vi "STICK_house.vi"() -> ()   [LabVIEW 2014]
panel:
  out "Temperature in Volts [V]":dbl format="%#_4g"
  out "On/Off":bool
  out "Error out":errorcluster
  out "P1":T1
  out "P2":T2
  out "Device ID":string
  in  "VISA resource name":refnum<visa-resource-name>
  out "Error":bool
  in  "Thermostat ON/OFF":bool=TRUE
  out "Happiness [%]":dbl(slide) scale=0.0..100.0
  out "Status":string="Water frozen!"
  out "Thermostat [°C]":dbl=20.0
  out "Outdoor temp":dbl(slide) scale=-20.0..40.0
  out "Time":timestamp format="%<%H:%M>T"
  out "Boiler temp":dbl(knob) max=60.0 scale=0.0..100.0
  out "Room temp":dbl(slide) scale=0.0..40.0
  out "Room [°C]":dbl format="%#_3g"
  out "Heat":bool
  out "?":T3(graph)
  in  "Stop Button":bool
  # "System values"
  # "Thermostat"
  # "Boiler"
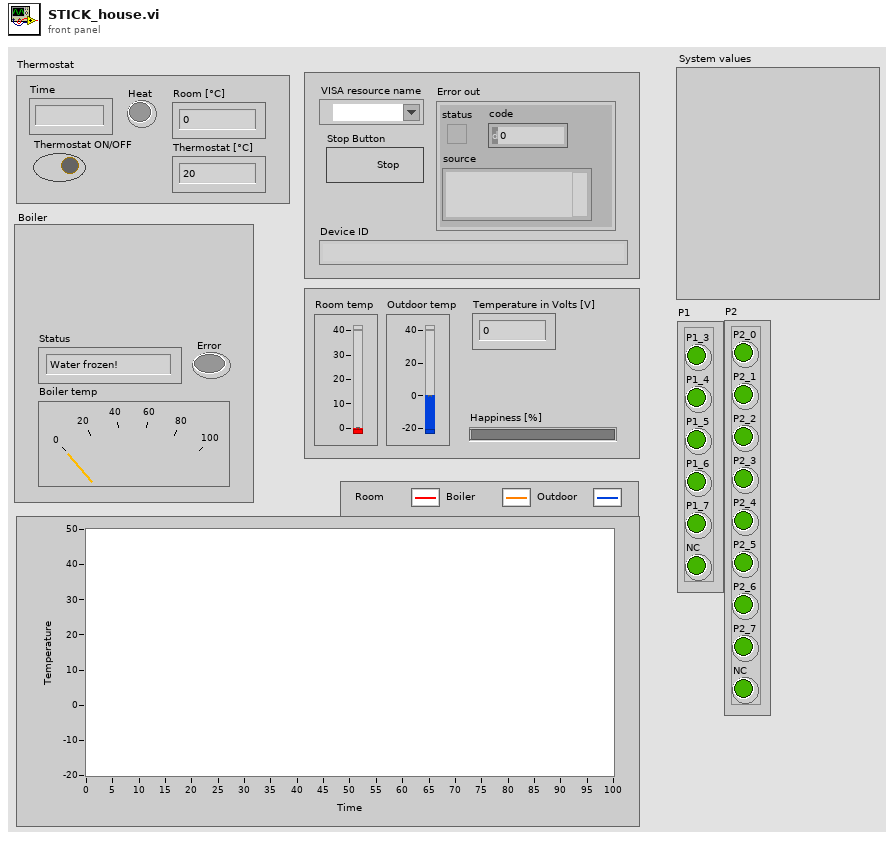
[diagram p1: front panel]
types:
  T1 = cluster{"P1_0":bool, "P1_1":bool, "P1_2":bool, "P1_3":bool, "P1_4":bool, "P1_5":bool, "P1_6":bool, "P1_7":bool, "NC":bool}
  T2 = cluster{"P2_0":bool, "P2_1":bool, "P2_2":bool, "P2_3":bool, "P2_4":bool, "P2_5":bool, "P2_6":bool, "P2_7":bool, "NC":bool}
  T3 = cluster{"T_room":dbl, "T_heater":dbl, "temp out":dbl}
  T4 = cluster{"T_room":dbl, "T_heater":dbl, "temp out":dbl}[]
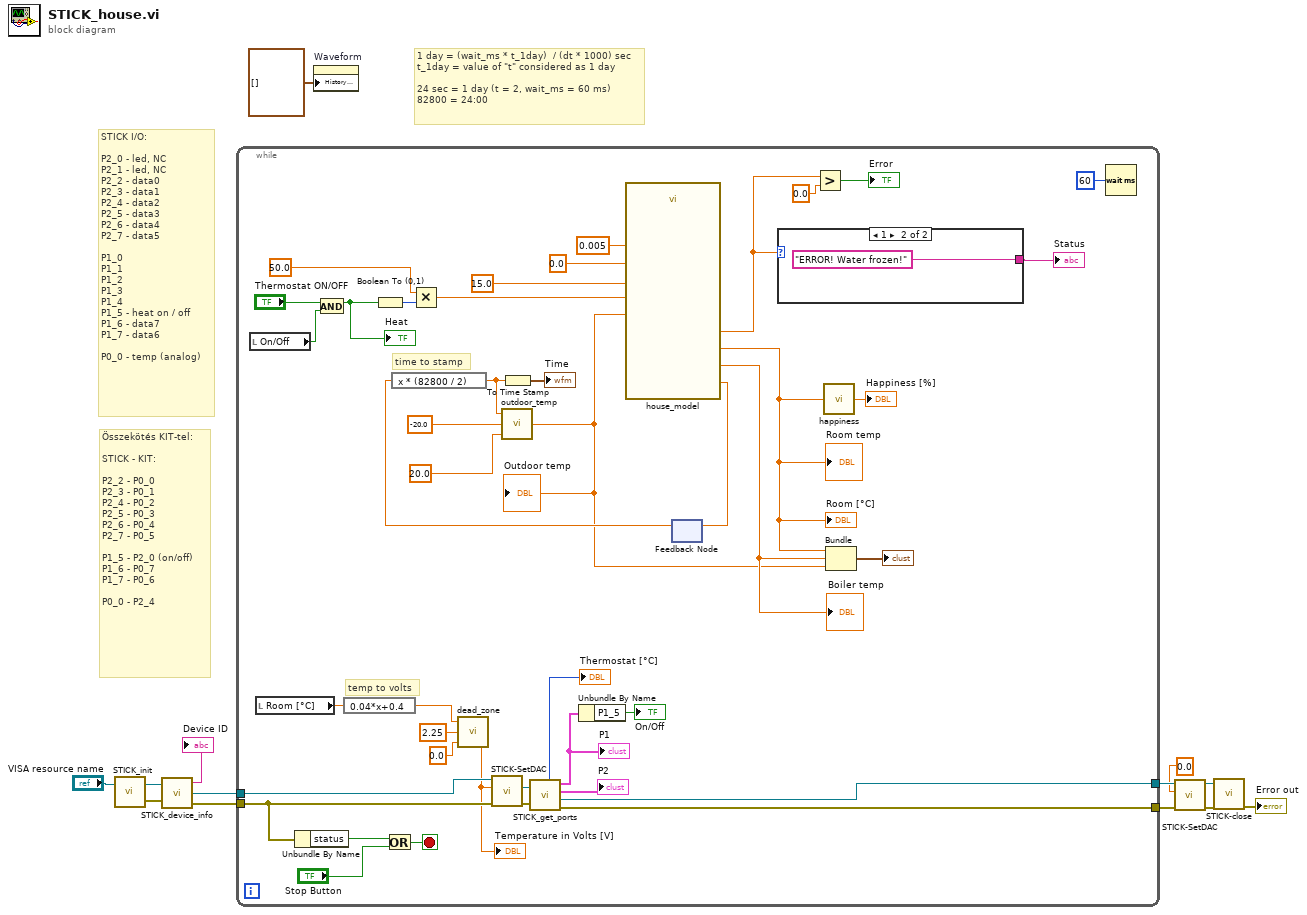
[diagram p0: block diagram]
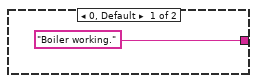
[diagram p2: hidden frame]
diagram:
  # "Összekötés KIT-tel:\n\nSTICK - KIT:\n\nP2_2 - P0_0\nP2_3 - P0_1\nP2_4 - P0_2\nP2_5 - P0_3\nP2_6 - P0_4\nP2_7 - P0_5\n\nP1_5 - P2_0 (on/off)\nP1_6 - P0_7\nP1_7 - P0_6\n\nP0_0 - P2_4"
  # "STICK I/O:\n\nP2_0 - led, NC\nP2_1 - led, NC\nP2_2 - data0\nP2_3 - data1\nP2_4 - data2\nP2_5 - data3\nP2_6 - data4\nP2_7 - data5\n\nP1_0 \nP1_1\nP1_2\nP1_3\nP1_4\nP1_5 - heat on / off\nP1_6 - data7\nP1_7 - data6\n\nP0_0 - temp (analog)"
  # "1 day = (wait_ms * t_1day)  / (dt * 1000) sec\nt_1day = value of \"t\" considered as 1 day\n\n24 sec = 1 day (t = 2, wait_ms = 60 ms)\n82800 = 24:00"
  n1 = call "STICK_init.vi"("VISA Refnum in"="VISA resource name") -> ("error out"=w11:errorcluster, "VISA Refnum out"=w10:refnum<visa-resource-name>)  [unwired: 1 in]
  n2 = call "STICK_device_info.vi"("VISA Refnum in"=w10, "error in (no error)"=w11) -> ("read buffer"=→"Device ID":string, "VISA Refnum out"=w1:refnum<visa-resource-name>, "error out"=w2:errorcluster)
  n3 = while {
    tunnel: [w27] -> w5
    tunnel: [w26] -> w3
    tunnel: w2 -> [w24]
    tunnel: w1 -> [w25]
    stop <- w31 stop-if-true
    # "time to stamp"
    # "temp to volts"
    n4 = local read "On/Off"() -> (w20:bool)
    n5 = local read "Room [°C]"() -> (w22:dbl)
    n6 = Unbundle By Name(w24) -> ("status"=w23:bool)
    n7 = And(x="Thermostat ON/OFF", y=w20) -> (x .and. y?=w36:bool)
    "Heat" <- w36
    n8 = expression code="0.04*x+0.4"(w22) -> (w15:dbl)
    n9 = Boolean To (0,1)(Boolean=w36) -> (0, 1=w55:i16)
    n10 = Or(x=w23, y="Stop Button") -> (x .or. y?=w31:bool)
    n11 = Multiply(x=50.0 ("Heater temp [°C]"), y=w55) -> (x*y=w54:dbl)
    n12 = call "dead_zone.vi"("min"=0.0, "max"=2.25, "number in"=w15) -> ("number out"=w14:dbl)
    "Temperature in Volts [V]" <- w14
    n13 = call "STICK-SetDAC.vi"("error in (no error)"=w24, "IDA 0 [V]"=w14, "VISA resource name"=w25) -> ("error out"=w29:errorcluster, "VISA resource name out"=w28:refnum<visa-resource-name>)  [unwired: 3 in]
    n14 = call "STICK_get_ports.vi"("error in (no error)"=w29, "VISA Refnum in"=w28) -> ("error out"=w26:errorcluster, "VISA Refnum out"=w27:refnum<visa-resource-name>, "P2"=→"P2":T2, "P1"=w33:T1, "data"=→"Thermostat [°C]":u8)
    "P1" <- w33
    n15 = Unbundle By Name(w33) -> ("P1_5"=→"On/Off":bool)
    n16 = feedback #1() -> (w42:dbl)  [unwired: 1 in]
    n17 = expression code="x * (82800 / 2)"(w42) -> (w52:dbl)
    n18 = call "outdoor_temp.vi"("temp max"=20.0 ("Temp max"), "temp min"=-20.0 ("Temp min"), "time in"=w52) -> ("temp out"=w39:dbl)
    "Outdoor temp" <- w39
    n19 = To Time Stamp(1:w52) -> (0:→"Time":timestamp)
    n20 = call "house_model.vi"("T_out"=w39, "dt"=0.005, "t_0"=0.0 ("t"), "T_room_0"=15.0 ("T_room_0 [°C]"), "heat_level"=w54) -> ("T_room"=w34:dbl, "error_code"=w47:dbl, "t"=w40:dbl, "T_heater"=w44:dbl)  [unwired: 5 in, 2 out]
    "Room [°C]" <- w34
    "Room temp" <- w34
    "Boiler temp" <- w44
    n21 = feedback-in #1(w40) -> ()
    n22 = case shown="1" w47 {
      tunnel: ["Boiler working." "ERROR! Water frozen!"] -> w35
      frame 0, Default {
      }
      frame 1 {
      }
    }
    "Status" <- w35
    n23 = Greater?(x=w47, y=0.0) -> (0:→"Error":bool)
    n24 = call "happiness.vi"("T_room"=w34) -> ("Happiness [%]"=→"Happiness [%]":dbl)
    n25 = Bundle("T_room"=w34, "T_heater"=w44, "temp out"=w39) -> (→"?":T3)  [unwired: 1 in]
    n26 = Wait (ms)(milliseconds to wait=u32 60) -> ()  [unwired: 1 out]
  }
  n27 = property on="Waveform" class="WFChart (strict)"("History Data"=T4 []) -> ()  [unwired: 2 in, 2 out]
  n28 = call "STICK-SetDAC.vi"("error in (no error)"=w3, "IDA 0 [V]"=0.0 ("DAC  1 [V]"), "VISA resource name"=w5) -> ("error out"=w7:errorcluster, "VISA resource name out"=w6:refnum<visa-resource-name>)  [unwired: 3 in]
  n29 = call "STICK-close.vi"("error in (no error)"=w7, "VISA resource name"=w6) -> ("error out"=→"Error out":errorcluster)  [unwired: 4 in, 1 out]
